vi "Kinect Extract Mouse.vi"(0 "Particle Report":T2, 5 "Image Src":T1, 7 "Image Mask":T1, 9 "Image Dst":T1, 11 "error in (no error)":errorcluster) -> (4 "Cropped Image Out":T1, 15 "error out":errorcluster)   [LabVIEW 2011]
uses:
  <vilib>/vision/Image Controls.llb/IMAQ Image.ctl
  <vilib>/vision/NI_Vision_Development_Module.lvlib
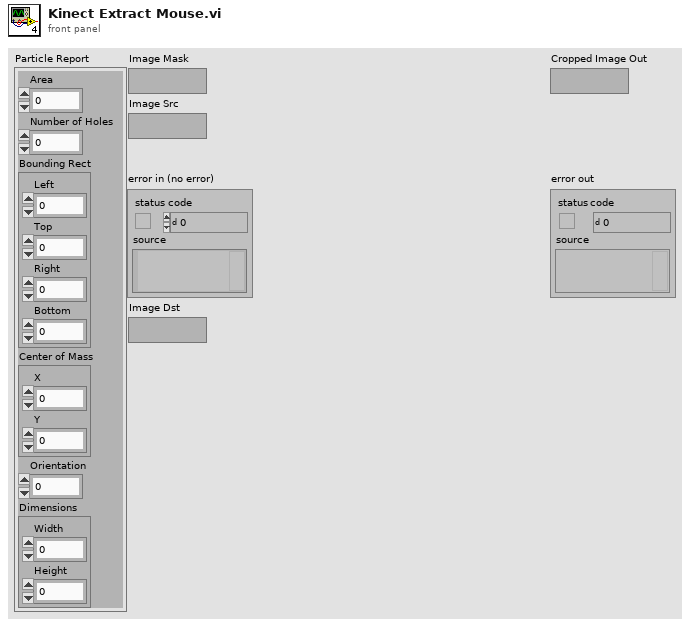
[diagram p1: front panel]
types:
  T1 = typedef "IMAQ Image.ctl" = refnum<image>
  T2 = cluster{"Area":dbl, "Number of Holes":dbl, "Bounding Rect":cluster{"Left":dbl, "Top":dbl, "Right":dbl, "Bottom":dbl}, "Center of Mass":cluster{"X":dbl, "Y":dbl}, "Orientation":dbl, "Dimensions":cluster{"Width":dbl, "Height":dbl}}
  T3 = cluster{"Left":dbl, "Top":dbl, "Right":dbl, "Bottom":dbl}
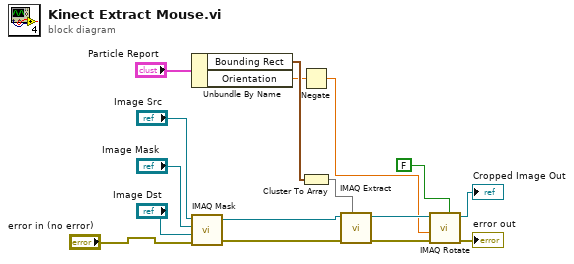
[diagram p0: block diagram]
diagram:
  n1 = Unbundle By Name("Particle Report") -> ("Bounding Rect"=w15:T3, "Orientation"=w11:dbl)
  n2 = call "IMAQ Mask"("error in (no error)"="error in (no error)", "Image Dst"="Image Dst", "Image Mask"="Image Mask", "Image Src"="Image Src") -> ("error out"=w5:errorcluster, "Image Dst Out"=w16:T1)  [unwired: 1 in]
  n3 = Negate(x=w11) -> (-x=w10:dbl)
  n4 = Cluster To Array(cluster=w15) -> (array=w14:dbl[])
  n5 = call "IMAQ Extract"("Optional Rectangle"=w14, "error in (no error)"=w5, "Image Src"=w16) -> ("error out"=w4:errorcluster, "Image Dst Out"=w13:T1)  [unwired: 7 in]
  n6 = call "IMAQ Rotate"("Maintain Size"=FALSE, "error in (no error)"=w4, "Angle (degrees)"=w10, "Image Src"=w13) -> ("error out"=→"error out":errorcluster, "Image Dst Out"=→"Cropped Image Out":T1)  [unwired: 6 in]
